vi "1.0.0_Initialisation.vi"(6 ".bat":T1={"getVersion"="Getting Software Version.bat", "Start Test mode"="Start Test Mode.bat", "Start camera test mode"="Start camera test mode.bat", "get one RAW Image"="Get one image.bat", "Stop camera test mode"="Stop camera test mode.bat", "Stop Test Mode"="Stop Test Mode.bat", "Get image reflection"="Get image reflection.bat", "Get image uniformity andFlash LED brightness"="Get image uniformity andFlash LED brightness.bat", "Disable flash LED"="Disable flash LED.bat", "Enable flash LED"="Enable flash LED.bat", "Software Reset"="Software Reset.bat", "Tune Flash LED brightness"="Tune Flash LED brightness.bat", "Start Camera calibration"="Start Camera calibration.bat", "Verify OBC Setting"="Verify OBC Setting.bat"}, 7 "Data in":T2, 8 "error in (no error)":errorcluster, 9 "AllControls In":T3, 11 "Message Queue out":T4) -> (0 "error out":errorcluster, 1 "Flow":string, 3 "Message Queue Out":T4, 5 "Data out":T2)   [LabVIEW 2017]
uses:
  Depends/AMC/subVIs/TypeDefs/amc_Message Queue.ctl
  Depends/AMC/subVIs/TypeDefs/amc_Message.ctl
  Depends/Tools/Keyed Array/Tools_KeyedArray KeyedArray.ctl
  Ctrls/AllControls.ctl
  Ctrls/CSV_Data.ctl
  Ctrls/NFC.bat
panel:
  # "Start Test Mode/682_eol_cli_v02_004.exe -f test -p 1 -x nfc -c \nGetting Software Version/682_eol_cli_v02_004.exe -f version -t 0 -x nfc -c \nStart camera test mode/682_eol_cli_v02_004.exe -f camera -p 1 -x nfc -c \nGet one image/682_eol_cli_v02_004.exe -f camera -p2 -x nfc -c \nStop camera test mode/682_eol_cli_v02_004.exe -f camera -p0 -x nfc -c \nStop Test Mode/682_eol_cli_v02_004.exe -f test -p 0 -x nfc -c"
types:
  T1 = typedef "NFC.bat" = cluster{"getVersion":string, "Start Test mode":string, "Start camera test mode":string, "get one RAW Image":string, "Stop camera test mode":string, "Stop Test Mode":string, "Get image reflection":string, "Get image uniformity andFlash LED brightness":string, "Disable flash LED":string, "Enable flash LED":string, "Software Reset":string, "Tune Flash LED brightness":string, "Start Camera calibration":string, "Verify OBC Setting":string}
  T2 = typedef "CSV_Data.ctl" = cluster{"Version":cluster{"SC_Version":string, "VP_Version":string}, "SN":string, "Table":string[][], "Count":cluster{"Total":i32, "OK":i32, "NG":i32, "Yield":dbl}, "Start Time":timestamp, "daemon reference":refnum<k5>, "CT":dbl, "Config":string[][], "OK/NG":bool, "Station ID":string, "MES DDM SN":string, "MES PCBA SN":string, "Retest":string, "Lux":string, "VOT":cluster{"Initial brightness":string, "Mean uniformity":string, "Uniformity_Deviation":string, "Adjusted brightness":string, "Mean_Adjusted":string, "Deviation_Adjusted":string, "Reflection":string, "Result":bool}, "SKU":string, "Plate_Diameter":string, "Alarm":string}
  T3 = typedef "AllControls.ctl" = cluster{"MainVI":refnum<vi>, "AlarmInfo":refnum<vi>, "Log":refnum<vi>, "Current CT":refnum<vi>, "ProductID":refnum<vi>, "Device state":refnum<vi>, "MES":refnum<vi>, "mode":refnum<vi>, "TestInfo":refnum<vi>, "SubPnl":refnum<vi>, "Table":refnum<vi>, "MES bool":refnum<vi>, "TestMode":refnum<vi>, "Recipe":refnum<vi>, "Fail resume":refnum<vi>, "LogIn":refnum<vi>, "Start":refnum<vi>, "Maintenance":refnum<vi>, "Stop":refnum<vi>, "Exit":refnum<vi>}
  T4 = typedef "amc_Message Queue.ctl" = refnum<queue>
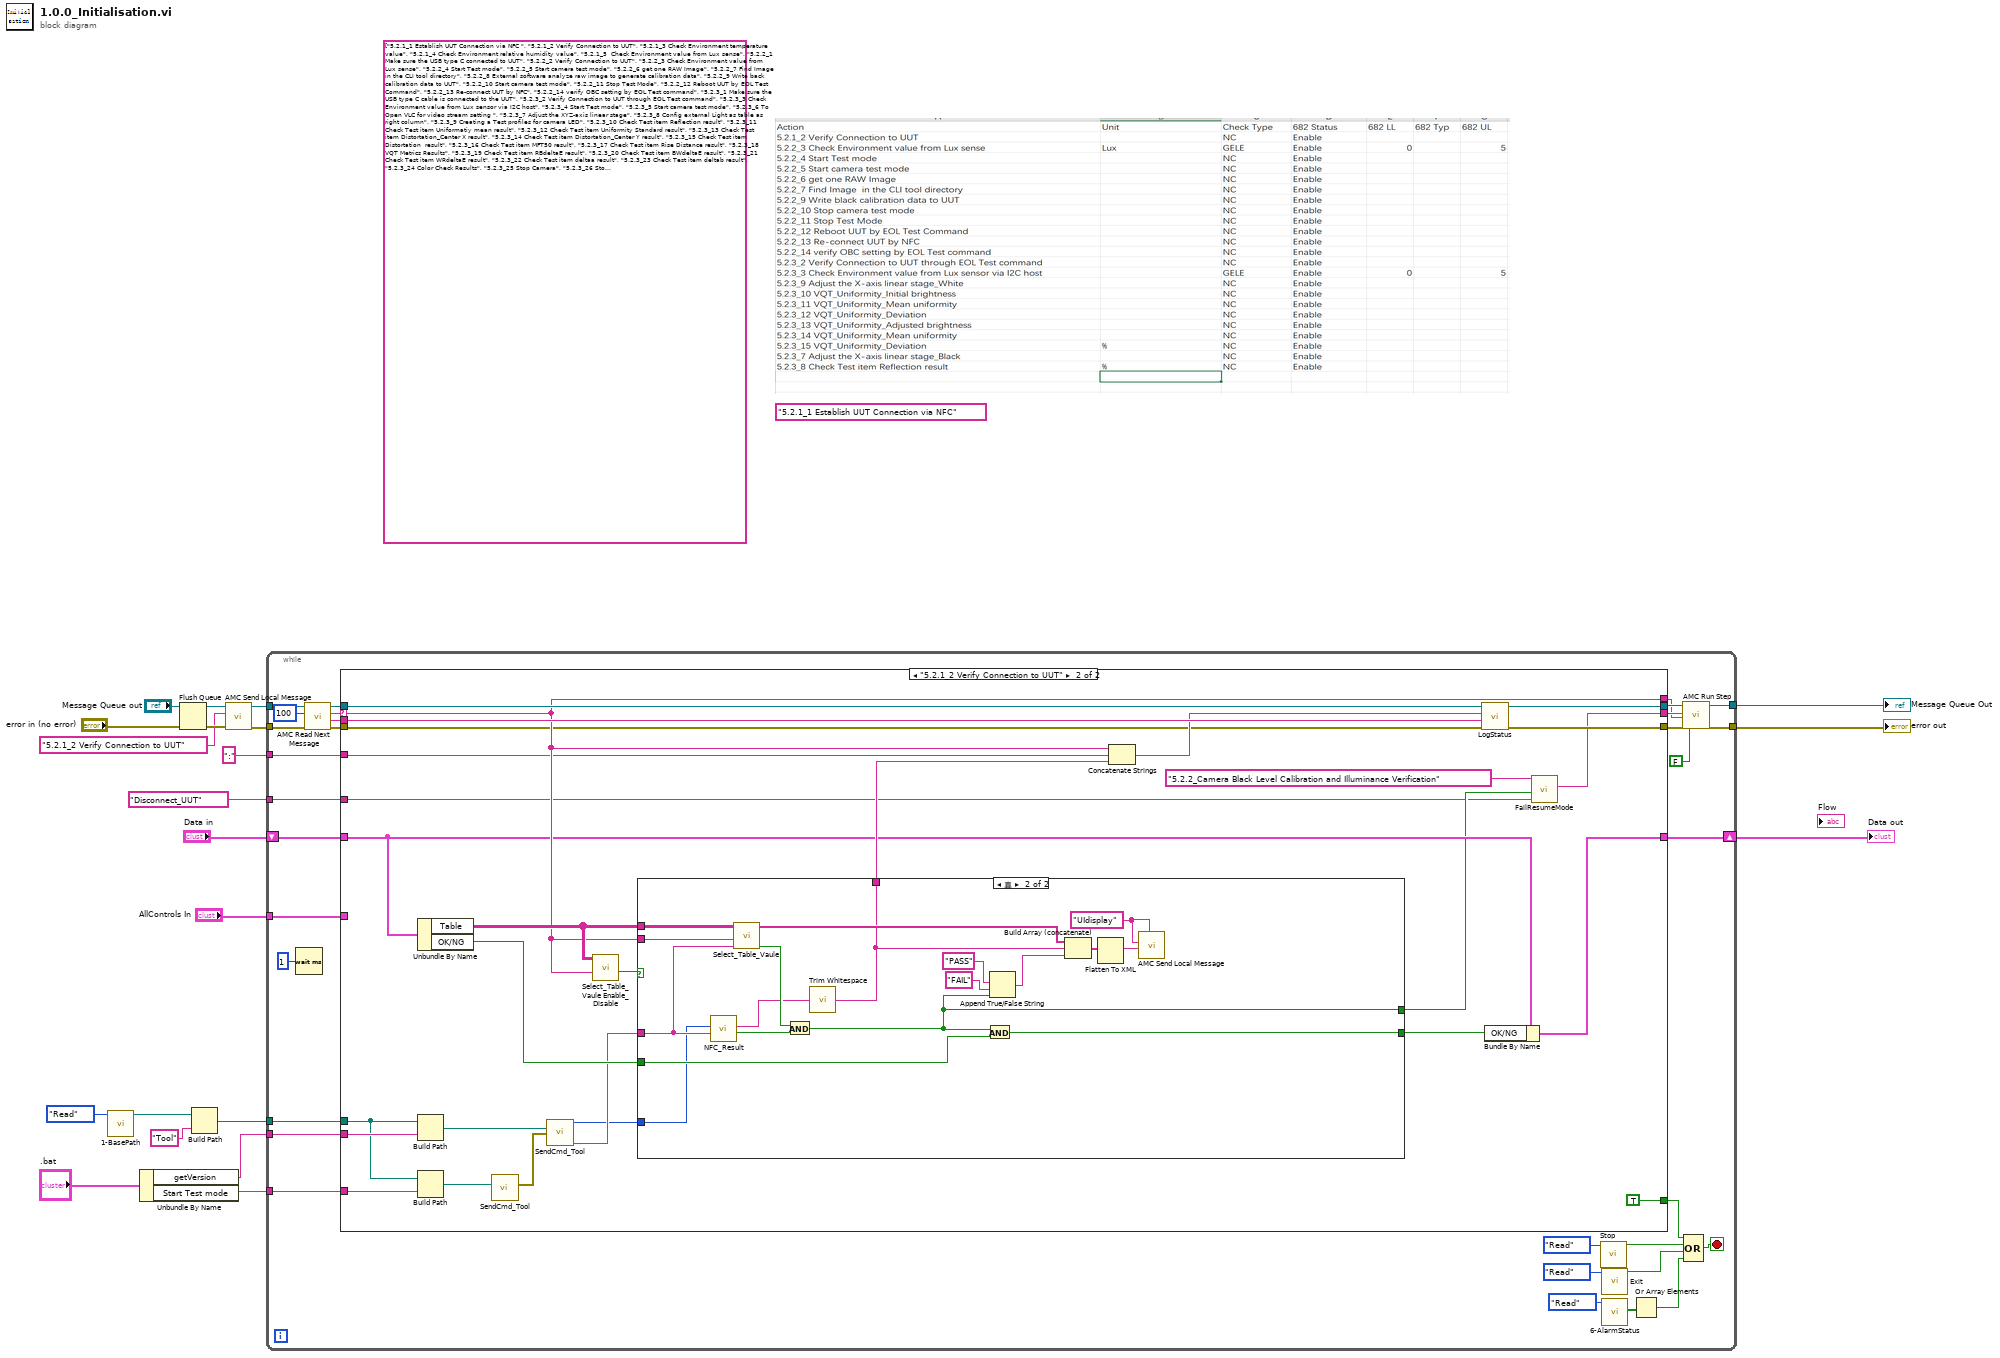
[diagram p0: block diagram]
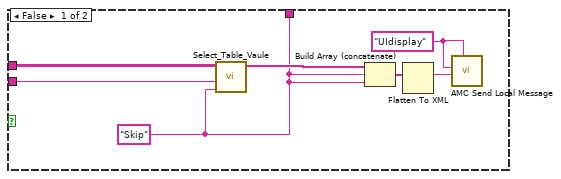
[diagram p3: hidden frame]
diagram:
  (unwired) string[] ["5.2.1_1 Establish UUT Connection via NFC ", "5.2.1_2 Verify Connection to UUT", "5.2.1_3 Check Environment temperature value", "5.2.1_4 Check Environment relative humidity value", "5.2.1_5  Check Environment value from Lux sense", "5.2.2_1 Make sure the USB type C connected to UUT", "5.2.2_2 Verify Connection to UUT", "5.2.2_3 Check Environment value from Lux sense", "5.2.2_4 Start Test mode", "5.2.2_5 Start camera test mode", "5.2.2_6 get one RAW Image", "5.2.2_7 Find Image  in the CLI tool directory", "5.2.2_8 External software analyze raw image to generate calibration data", "5.2.2_9 Write back calibration data to UUT", "5.2.2_10 Start camera test mode", "5.2.2_11 Stop Test Mode", "5.2.2_12 Reboot UUT by EOL Test Command", "5.2.2_13 Re-connect UUT by NFC", "5.2.2_14 verify OBC setting by EOL Test command", "5.2.3_1 Make sure the USB type C cable is connected to the UUT", "5.2.3_2 Verify Connection to UUT through EOL Test command", "5.2.3_3 Check Environment value from Lux sensor via I2C host", "5.2.3_4 Start Test mode", "5.2.3_5 Start camera test mode", "5.2.3_6 To Open VLC for video stream setting ", "5.2.3_7 Adjust the XYZ-axis linear stage", "5.2.3_8 Config external Light as table as right column", "5.2.3_9 Creating a Test profiles for camera LED", "5.2.3_10 Check Test item Reflection result", "5.2.3_11 Check Test item Uniformatiy mean result", "5.2.3_12 Check Test item Uniformity Standard result", "5.2.3_13 Check Test item Distortation_Center X result", "5.2.3_14 Check Test item Distortation_Center Y result", "5.2.3_15 Check Test item Distortation  result", "5.2.3_16 Check Test item MFT50 result", "5.2.3_17 Check Test item Rise Distance result", "5.2.3_18 VQT Metrics Results", "5.2.3_19 Check Test item RBdeltaE result", "5.2.3_20 Check Test item BWdeltaE result", "5.2.3_21 Check Test item WRdeltaE result", "5.2.3_22 Check Test item deltaa result", "5.2.3_23 Check Test item deltab result", "5.2.3_24 Color Check Results", "5.2.3_25 Stop Camera", "5.2.3_26 Stop Test mode", "5.2.3_27 Shutdown UUT"] ("subarray")
  (unwired) "5.2.1_1 Establish UUT Connection via NFC" ("Message Name")
  n1 = call "1-BasePath.vi"("Step"=enum16{"Initial", "Write", "Read"}."Read") -> ("Path Out"=w7:path)  [unwired: 9 in, 1 out]
  n2 = Unbundle By Name(".bat") -> ("getVersion"=w5:string, "Start Test mode"=w2:string)
  n3 = Flush Queue(queue="Message Queue out") -> (queue out=w16:T4)  [unwired: 1 in, 2 out]
  n4 = Build Path(base path=w7, name or relative path="Tool") -> (appended path=w6:path)
  n5 = call "AMC Send Local Message.vi"("error in (no error)"="error in (no error)", "Message Name"="5.2.1_2 Verify Connection to UUT", "Message Queue in"=w16) -> ("error out"=w18:errorcluster, "Message Queue out"=w19:T4)  [unwired: 7 in]
  n6 = while {
    tunnel: w19 -> [w52]
    tunnel: [w48] -> w15
    tunnel: w18 -> [w46]
    tunnel: [w43] -> w14
    tunnel: "AllControls In" -> [w31]
    shift-right: [w29] -> w11
    shift-left: "Data in" -> [w30]
    tunnel: w6 -> [w25]
    tunnel: w5 -> [w24]
    tunnel: ":" -> [w23]
    tunnel: "Disconnect_UUT" -> [w22]
    tunnel: w2 -> [w21]
    stop <- w34 stop-if-true
    n7 = Wait (ms)(milliseconds to wait=u32 1 ("等待时间（毫秒）")) -> ()  [unwired: 1 out]
    n8 = call "AMC Read Next Message.vi"("error in (no error)"=w46, "timeout (1ms)"=100, "Message Queue in"=w52) -> ("error out"=w45:errorcluster, "Message Value"=w39:string, "Message Name"=w50:string, "Message Queue out"=w51:T4)  [unwired: 1 in, 4 out]
    n9 = case shown="\"5.2.1_2 Verify Connection to UUT\"" w50 {
      selector: w50 -> [_ w77]
      tunnel: w51 -> [w55 w82]
      tunnel: [w55 w82] -> w49
      tunnel: w45 -> [w54 w76]
      tunnel: [w54 w81] -> w44
      tunnel: [_ TRUE ("GRR")] -> w35
      tunnel: w39 -> [_ w80]
      tunnel: [_ w77] -> w38
      tunnel: [_ w61] -> w40
      tunnel: w31 -> [_ _]
      tunnel: w30 -> [w53 w73]
      tunnel: [w53 w72] -> w29
      tunnel: w25 -> [_ w59]
      tunnel: w24 -> [_ w69]
      tunnel: w23 -> [_ w65]
      tunnel: w22 -> [_ w60]
      tunnel: w21 -> [_ w58]
      frame "假", Default {
      }
      frame "5.2.1_2 Verify Connection to UUT" {
        n10 = Build Path(base path=w59, name or relative path=w69) -> (appended path=w68:path)
        n11 = Build Path(base path=w59, name or relative path=w58) -> (appended path=w57:path)
        n12 = Unbundle By Name(w73) -> ("Table"=w78:string[][], "OK/NG"=w70:bool)
        n13 = call "SendCmd_Tool.vi"("path_bat"=w57) -> ("error out 3"=w56:errorcluster)  [unwired: 7 in, 7 out]
        n14 = call "SendCmd_Tool.vi"("path_bat"=w68, "error in (no error) 2"=w56) -> ("return code"=w66:i32, "version info"=w67:string)  [unwired: 6 in, 6 out]
        n15 = call "Select_Table_Vaule Enable_Disable.vi"("Action"=w77, "Table"=w78) -> ("Enable"=w74:bool)  [unwired: 8 in, 1 out]
        n16 = case shown="真" w74 {
          tunnel: [w83 w90] -> w75
          tunnel: w78 -> [w85 w101]
          tunnel: w77 -> [w84 w100]
          tunnel: w67 -> [_ w95]
          tunnel: [_ w96] -> w64
          tunnel: w70 -> [_ w97]
          tunnel: w66 -> [_ w93]
          tunnel: [_ w91] -> w62
          frame False {
            w89 = "UIdisplay" ("Process (\"\" - local)")
            w83 = "Skip" ("Action")
            n17 = call "Select_Table_Vaule.vi"("Vaule"=w83, "Action"=w84, "Table"=w85) -> ("vaule"=w86:string[])  [unwired: 7 in, 1 out]
            n18 = Build Array (concatenate)(w86, w83, w83) -> (w88:string[])
            n19 = Flatten To XML(anything=w88) -> (xml string=w87:string)
            n20 = call "AMC Send Local Message.vi"("Process (\"\" - local)"=w89, "Message Value"=w87, "Message Name"=w89) -> ()  [unwired: 7 in, 2 out]
          }
          frame True {
            w106 = "UIdisplay" ("Process (\"\" - local)")
            n21 = call "NFC_Result.vi"("input"=w95, "return code"=w93) -> ("Command Sucess"=w94:bool, "return_result"=w92:string)  [unwired: 8 in]
            n22 = call "Select_Table_Vaule.vi"("Vaule"=w95, "Action"=w100, "Table"=w101) -> ("Result"=w98:bool, "vaule"=w107:string[])  [unwired: 7 in]
            n23 = And(x=w98, y=w94) -> (x .and. y?=w91:bool)
            n24 = call <vilib>:"Trim Whitespace.vi"("string"=w92) -> ("trimmed string"=w90:string)  [unwired: 1 in]
            n25 = And(x=w91, y=w97) -> (x .and. y?=w96:bool)
            n26 = Append True/False String(1:w91, 2:"FAIL" ("真字符串"), 3:"PASS" ("真字符串")) -> (0:w99:string)  [unwired: 1 in]
            n27 = Build Array (concatenate)(w107, w90, w99) -> (w105:string[])
            n28 = Flatten To XML(anything=w105) -> (xml string=w104:string)
            n29 = call "AMC Send Local Message.vi"("Process (\"\" - local)"=w106, "Message Value"=w104, "Message Name"=w106) -> ()  [unwired: 7 in, 2 out]
          }
        }
        n30 = Concatenate Strings(w77, w65, w75) -> (w79:string)
        n31 = call "LogStatus.vi"("error in (no error)"=w76, "last message"=w80, "message"=w79) -> ("error  out"=w81:errorcluster)  [unwired: 8 in]
        n32 = Bundle By Name(cluster=w73, "OK/NG"=w64) -> (w72:T2)
        n33 = call "FailResumeMode.vi"("NextMessage"="5.2.2_Camera Black Level Calibration and Illuminance Verification", "OK/NG"=w62, "EndMessage"=w60) -> ("OutMessage"=w61:string)  [unwired: 6 in]
      }
    }
    n34 = call "Stop.vi"("Step"=enum16{"Initial", "Write", "Read"}."Read") -> ("Stop Out"=w33:bool)  [unwired: 9 in, 1 out]
    n35 = call "Exit.vi"("Step"=enum16{"Initial", "Write", "Read"}."Read" ("step")) -> ("Exit Out"=w32:bool)  [unwired: 9 in, 1 out]
    n36 = call "6-AlarmStatus.vi"("Step"=enum16{"Initial", "Write", "Read"}."Read") -> ("AlarmValue Out"=w27:bool[])  [unwired: 9 in, 1 out]
    n37 = Or Array Elements(Boolean array=w27) -> (logical OR=w26:bool)
    n38 = call "AMC Run Step.vi"("Message Queue In"=w49, "Message Name"=w40, "Message Value"=w38, "error in (no error)"=w44, "Mli/Sig"=FALSE) -> ("Message Queue Out"=w48:T4, "error out"=w43:errorcluster)  [unwired: 13 in]
    n39 = Compound Arithmetic op=OR(w35, w33, w32, w26) -> (w34:bool)
  }
  "Message Queue Out" <- w15
  "error out" <- w14
  "Data out" <- w11
